vi "round_buoy_details.vi"(8 "error in (no error)":errorcluster, 11 "Mission in":refnum<class "Mission.lvclass">) -> (0 "error out":errorcluster, 1 "Buoy to Round":cluster{"X":dbl, "Y":dbl}, 3 "Mission out":refnum<class "Mission.lvclass">)   [LabVIEW 2011, in "Mission.lvclass"]
uses:
  Mission.lvclass
  Mission.lvclass/Mission.ctl
panel:
  out "String":string
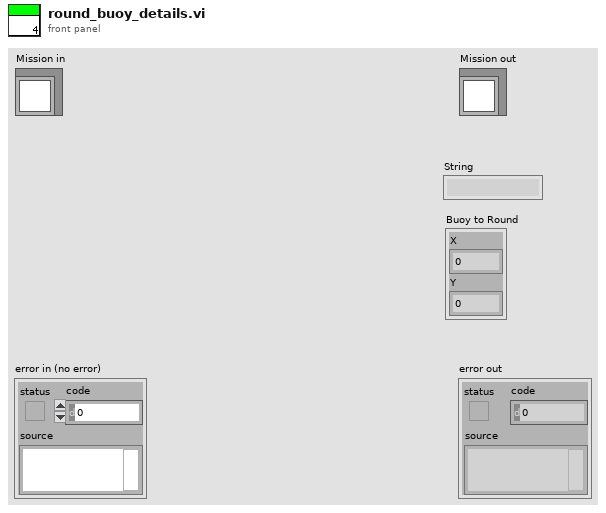
[diagram p1: front panel]
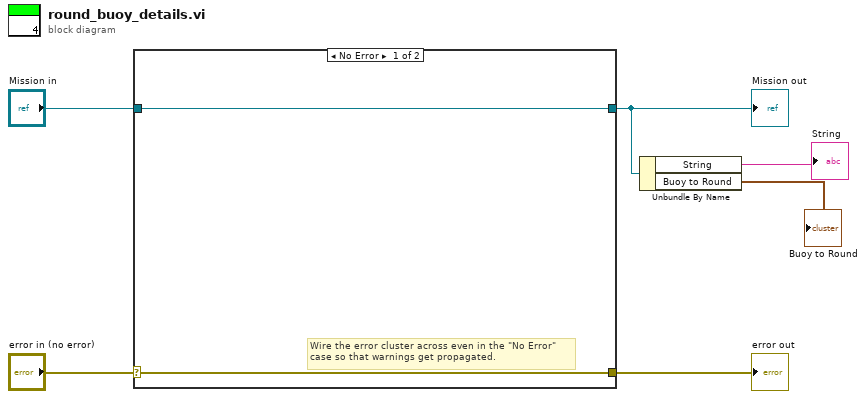
[diagram p0: block diagram]
diagram:
  n1 = case shown="No Error" "error in (no error)" {
    selector: "error in (no error)" -> [w7 w10]
    tunnel: [w7 w10] -> w5
    tunnel: [w8 w9] -> w3
    tunnel: "Mission in" -> [w8 w9]
    frame No Error {
      # "Wire the error cluster across even in the \"No Error\"\ncase so that warnings get propagated."
    }
    frame Error {
    }
  }
  "error out" <- w5
  "Mission out" <- w3
  n2 = Unbundle By Name(w3) -> ("String"=→"String":string, "Buoy to Round"=→"Buoy to Round":cluster{"X":dbl, "Y":dbl})
